vi "Test_waitForCompletion_exitControl.vi"(8 "error in (no error)":errorcluster, 11 "waitComplete_Ctl":T1) -> (0 "error out":errorcluster, 2 "function return":i32, 3 "waitComplete_Ctl out":T1)   [LabVIEW 2018, in "SALLV_Test.lvlib"]
doc: "int Test_shm_waitForCompletion_exitControlLV(Test_waitCompleteLV *waitComplete_Ctl);"
uses:
  SALLV_Test.lvlib
  SALLV_Test.so
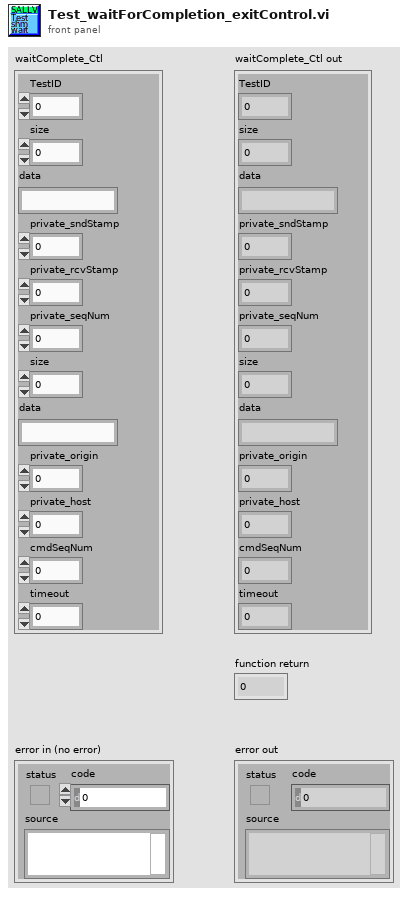
[diagram p1: front panel]
types:
  T1 = cluster{"TestID":i32, "size":i32, "data":string, "private_sndStamp":dbl, "private_rcvStamp":dbl, "private_seqNum":i32, "size":i32, "data":string, "private_origin":i32, "private_host":i32, "cmdSeqNum":i32, "timeout":u32}
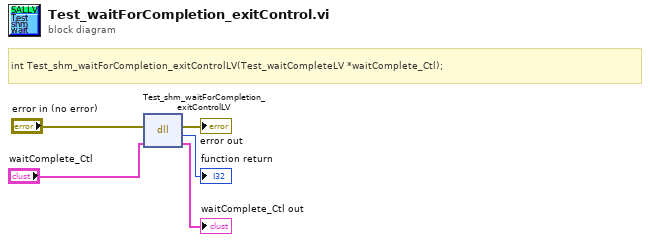
[diagram p0: block diagram]
diagram:
  # "int Test_shm_waitForCompletion_exitControlLV(Test_waitCompleteLV *waitComplete_Ctl);"
  n1 = dll-call lib="home/ttsai/Documents/github/ts_SALLabVIEW/testPerfTemp/TestData/SALLV_Test.*" fn="Test_shm_waitForCompletion_exitControlLV"(error in="error in (no error)", "waitComplete_Ctl"="waitComplete_Ctl") -> (error out=→"error out":errorcluster, →"function return":i32, "waitComplete_Ctl"=→"waitComplete_Ctl out":T1)  [unwired: 2 in, 1 out]
